vi "PrimaryInterfaceGetVariableValue.vi"(8 "Variable":refnum<k24>, 11 "error in":errorcluster) -> (0 "Value":T1, 3 "error out":errorcluster)   [LabVIEW 2023, in "UnderAutomation.UniversalRobots.lvlib"]
uses:
  UnderAutomation.UniversalRobots.lvlib
  C:/Users/fg/Documents/UniversalRobots.vi/UnderAutomation.UniversalRobots/lib/UnderAutomation.UniversalRobots.dll
  lib/UnderAutomation.UniversalRobots.dll
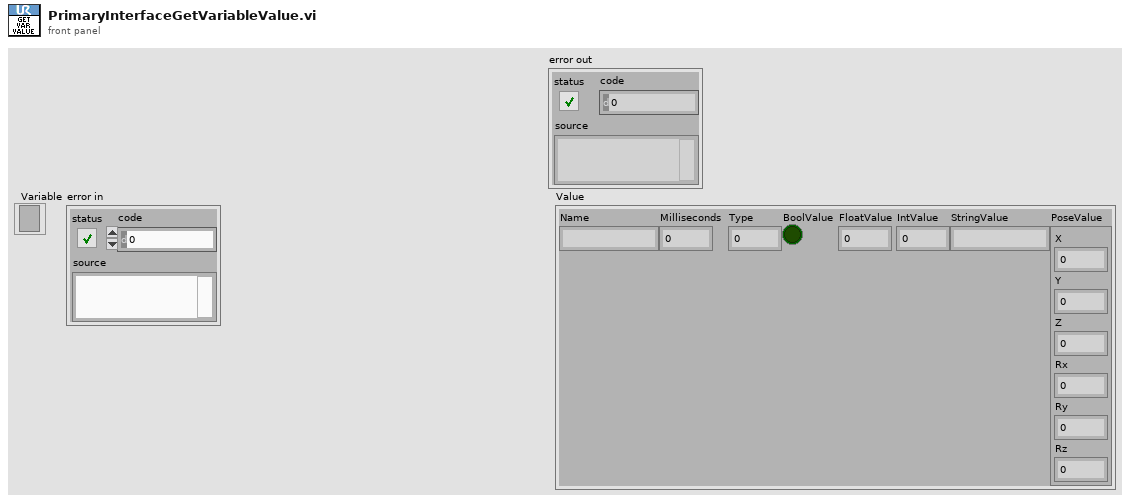
[diagram p1: front panel]
types:
  T1 = cluster{"Name":string, "Milliseconds":i32, "Type":i32, "BoolValue":bool, "FloatValue":sgl, "IntValue":i32, "StringValue":string, "PoseValue":cluster{"X":dbl, "Y":dbl, "Z":dbl, "Rx":dbl, "Ry":dbl, "Rz":dbl}}
  T2 = cluster{"X":dbl, "Y":dbl, "Z":dbl, "Rx":dbl, "Ry":dbl, "Rz":dbl}
  T3 = cluster{"Name":string, "Milliseconds":i32, "Type":i32, "ToBool":bool, "ToFloat":sgl, "ToInt":i32, "ToString":string, cluster{"X":dbl, "Y":dbl, "Z":dbl, "Rx":dbl, "Ry":dbl, "Rz":dbl}}
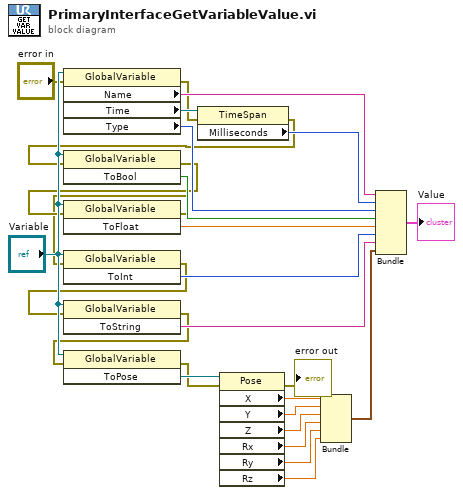
[diagram p0: block diagram]
diagram:
  n1 = property class="GlobalVariable"(reference="Variable", error in="error in") -> (error out=w8:errorcluster, "Name"=w15:string, "Time"=w13:refnum<k24>, "Type"=w14:i32)  [unwired: 1 out]
  n2 = property class="TimeSpan"(reference=w13, error in=w8) -> (error out=w7:errorcluster, "Milliseconds"=w12:i32)  [unwired: 1 out]
  n3 = invoke class="GlobalVariable" method="ToBool"(reference="Variable", error in=w7) -> (error out=w6:errorcluster, "ToBool"=w27:bool)  [unwired: 1 in, 1 out]
  n4 = invoke class="GlobalVariable" method="ToFloat"(reference="Variable", error in=w6) -> (error out=w5:errorcluster, "ToFloat"=w26:sgl)  [unwired: 1 in, 1 out]
  n5 = invoke class="GlobalVariable" method="ToInt"(reference="Variable", error in=w5) -> (error out=w4:errorcluster, "ToInt"=w17:i32)  [unwired: 1 in, 1 out]
  n6 = invoke class="GlobalVariable" method="ToString"(reference="Variable", error in=w4) -> (error out=w3:errorcluster, "ToString"=w18:string)  [unwired: 1 in, 1 out]
  n7 = invoke class="GlobalVariable" method="ToPose"(reference="Variable", error in=w3) -> (error out=w2:errorcluster, "ToPose"=w25:refnum<k24>)  [unwired: 1 in, 1 out]
  n8 = property class="Pose"(reference=w25, error in=w2) -> (error out=→"error out":errorcluster, "X"=w24:dbl, "Y"=w23:dbl, "Z"=w22:dbl, "Rx"=w21:dbl, "Ry"=w20:dbl, "Rz"=w19:dbl)  [unwired: 1 out]
  n9 = Bundle("X"=w24, "Y"=w23, "Z"=w22, "Rx"=w21, "Ry"=w20, "Rz"=w19) -> (w16:T2)  [unwired: 1 in]
  n10 = Bundle("Name"=w15, "Milliseconds"=w12, "Type"=w14, "ToBool"=w27, "ToFloat"=w26, "ToInt"=w17, "ToString"=w18, w16) -> (→"Value":T3)  [unwired: 1 in]
